vi "74HC194中的下降沿RS触发器.vi"(6 "R0":bool, 8 "R":bool, 9 "CP":bool, 11 "S":bool) -> (2 "Q":bool)   [LabVIEW 2018]
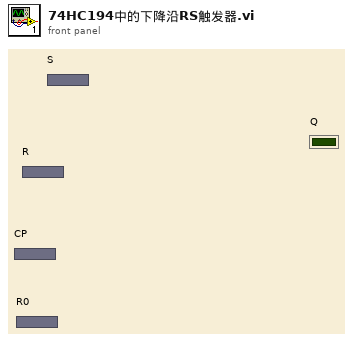
[diagram p1: front panel]
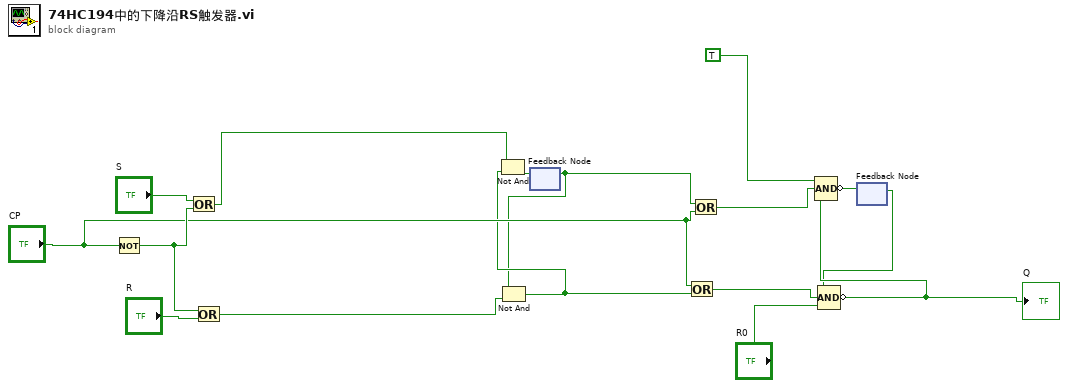
[diagram p0: block diagram]
diagram:
  n1 = Not(x="CP") -> (.not. x?=w11:bool)
  n2 = Or(x="S", y=w11) -> (x .or. y?=w14:bool)
  n3 = Or(x=w11, y="R") -> (x .or. y?=w12:bool)
  n4 = feedback #1() -> (w8:bool)  [unwired: 1 in]
  n5 = Not And(1:w12, 2:w8) -> (0:w9:bool)
  n6 = Not And(1:w9, 2:w14) -> (0:w16:bool)
  n7 = feedback-in #1(w16) -> ()
  n8 = Or(x="CP", y=w9) -> (x .or. y?=w6:bool)
  n9 = Or(x=w8, y="CP") -> (x .or. y?=w7:bool)
  n10 = feedback #2() -> (w3:bool)  [unwired: 1 in]
  n11 = Compound Arithmetic op=AND ("复合运算")(w3, w6, "R0") -> (invert w5:bool)
  "Q" <- w5
  n12 = Compound Arithmetic op=AND ("复合运算")(TRUE, w7, w5) -> (invert w4:bool)
  n13 = feedback-in #2(w4) -> ()
